vi "S8300E_reboot_UUT.vi"() -> ()   [LabVIEW 2011]
panel:
  out "Debug View":string
  out "VISA resource name out":refnum<visa-resource-name>
  out "進行狀況":string
  out "BEGIN TIME":u32
  # "2015-01-26"
  # "Error Code:MB-NG"
  # "S8300E REBOOT UUT"
  # "COM9 115200"
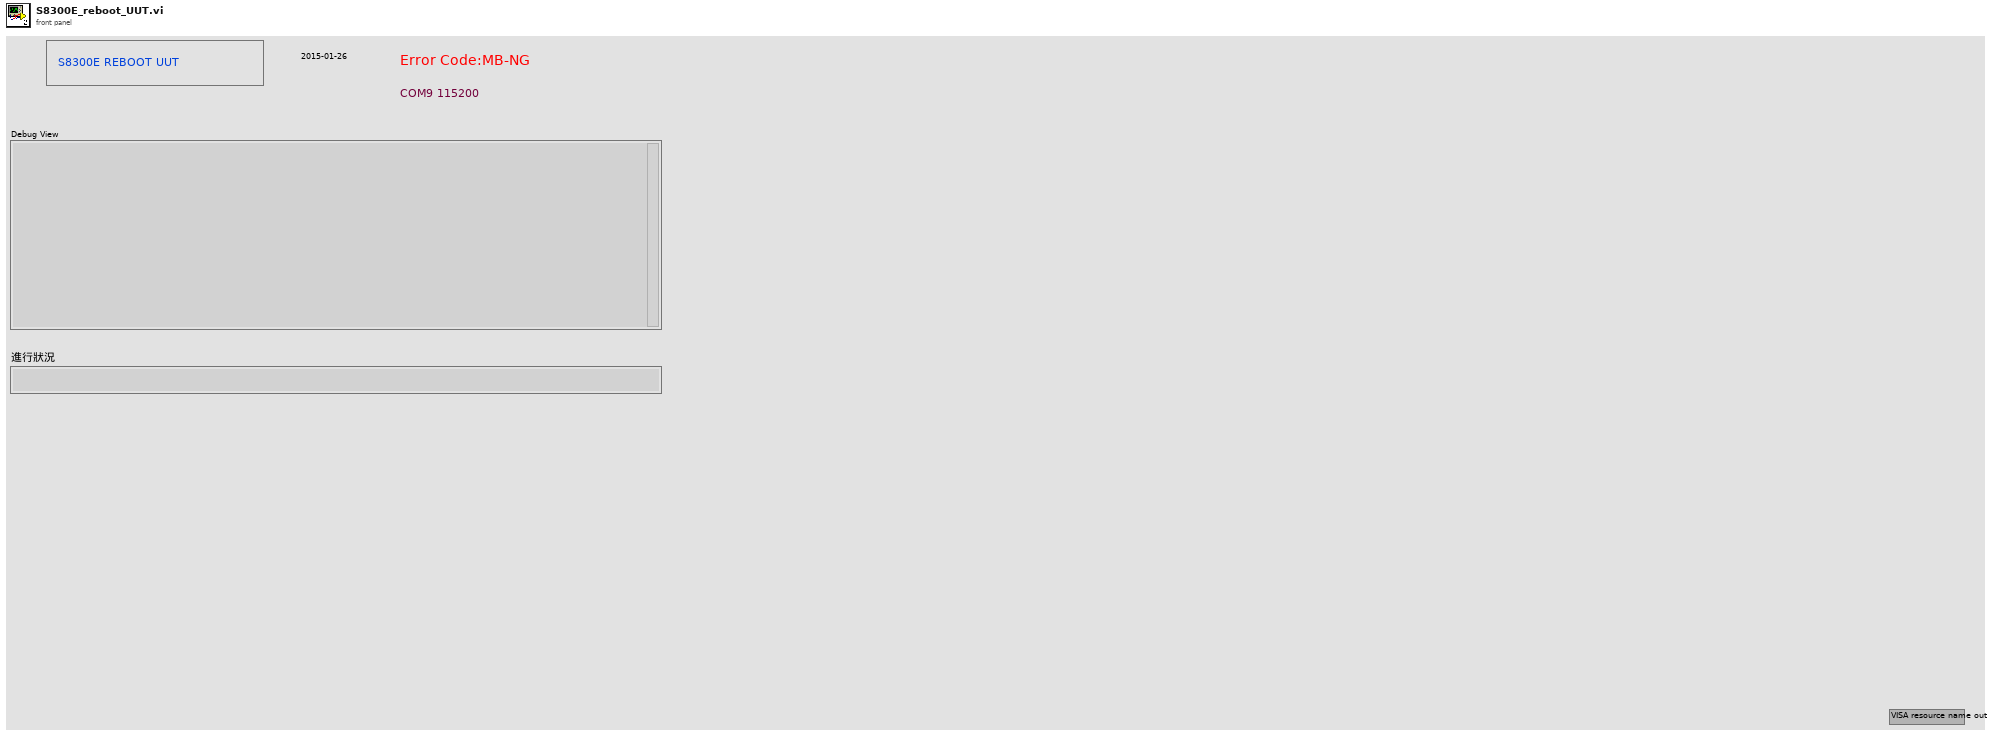
[diagram p1: front panel]
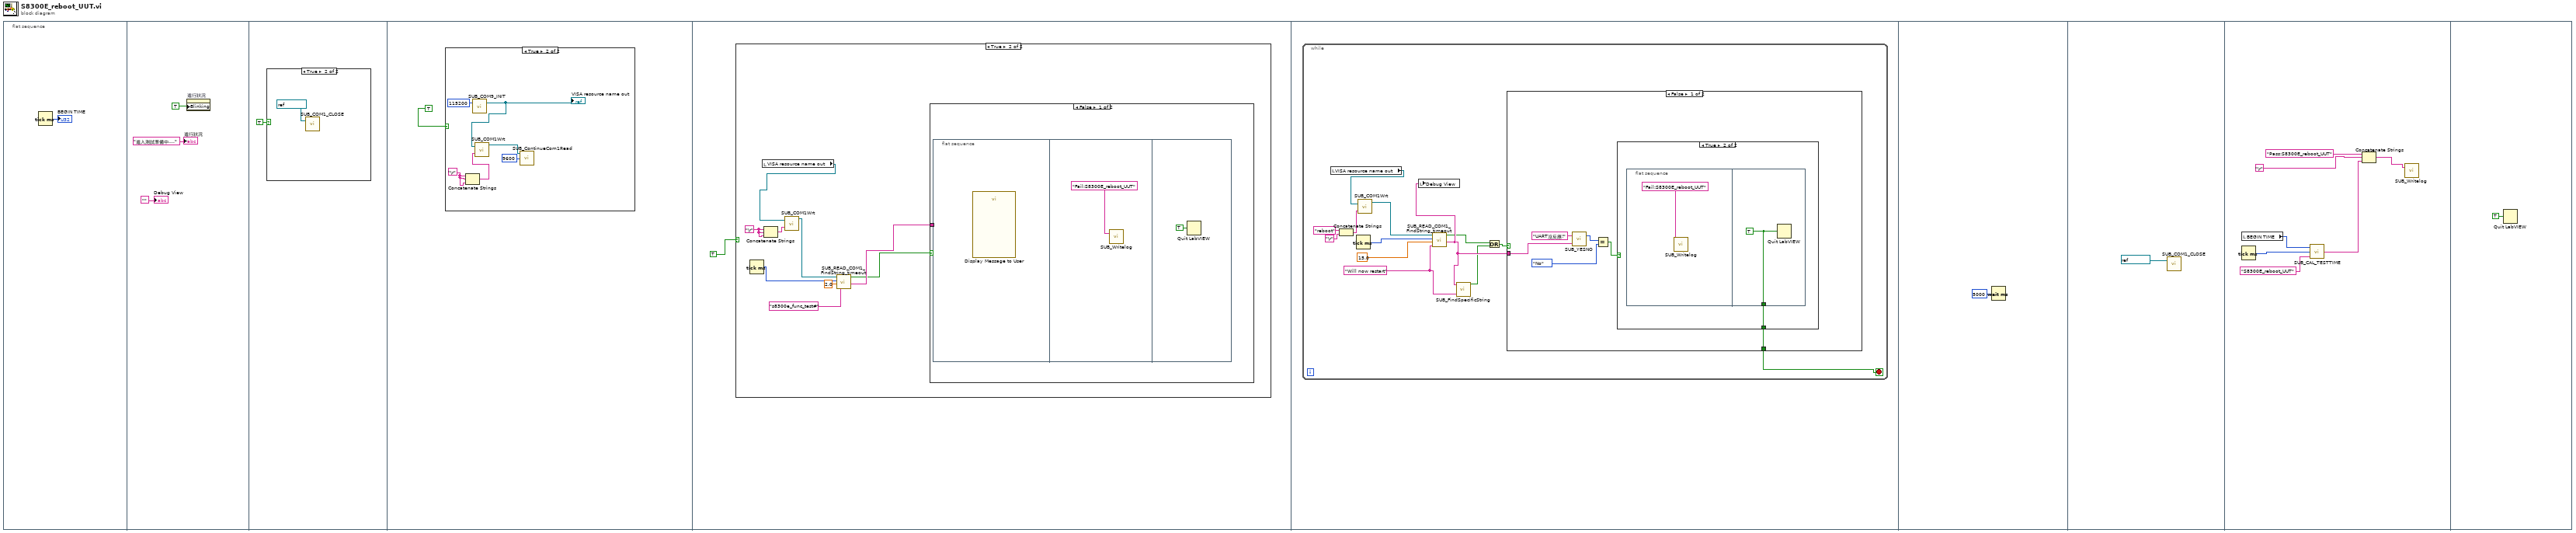
[diagram p0: block diagram]
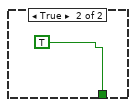
[diagram p7: hidden frame]
diagram:
  n1 = flat-sequence {
    frame #0 {
      n2 = Tick Count (ms)() -> (millisecond timer value=→"BEGIN TIME":u32)
    }
    frame #1 {
      n3 = property on="進行狀況" class="Str"("Blinking"=TRUE) -> ()  [unwired: 2 in, 2 out]
      "進行狀況" <- "進入測試準備中...." ("進行狀況")
      "Debug View" <- ""
    }
    frame #2 {
      n4 = case shown="True" TRUE {
        frame False {
        }
        frame True {
          n5 = call "SUB_COM1_CLOSE.vi"("VISA resource name"=refnum<visa-resource-name> "COM9") -> ()  [unwired: 3 in]
        }
      }
    }
    frame #3 {
      n6 = case shown="True" TRUE {
        frame False {
        }
        frame True {
          w9 = "\r"
          n7 = Concatenate Strings(w9, w9, w9) -> (w8:string)
          n8 = call "SUB_COM9_INIT.vi"("baud rate"=u32 115200) -> ("VISA resource name out"=w13:refnum<visa-resource-name>)  [unwired: 1 in, 1 out]
          "VISA resource name out" <- w13
          n9 = call "SUB_COM1Wrt.vi"("VISA resource name"=w13, "write buffer"=w8) -> ("duplicate VISA resource name"=w10:refnum<visa-resource-name>)  [unwired: 1 in, 1 out]
          n10 = call "SUB_ContinueCom1Read.vi"("Numeric"=9600, "duplicate VISA resource name 2"=w10) -> ()  [unwired: 1 in, 3 out]
        }
      }
    }
    frame #4 {
      n11 = case shown="True" TRUE {
        frame False {
        }
        frame True {
          w15 = "\r"
          n12 = Tick Count (ms)() -> (millisecond timer value=w20:u32)
          n13 = local read "VISA resource name out"() -> (w23:refnum<visa-resource-name>)
          n14 = Concatenate Strings(w15, w15, w15) -> (w16:string)
          n15 = call "SUB_COM1Wrt.vi"("VISA resource name"=w23, "write buffer"=w16) -> ("duplicate VISA resource name"=w21:refnum<visa-resource-name>)  [unwired: 1 in, 1 out]
          n16 = call "SUB_READ_COM1_FindString_timeout.vi"("Find this String"="s8300e_func_test#", "Timeout Seccond"=2.0, "Begin time"=w20, "duplicate VISA resource name 2"=w21) -> ("Output String"=w18:string, "Found String"=w17:bool)  [unwired: 1 in, 1 out]
          n17 = case shown="False" w17 {
            tunnel: w18 -> [_ _]
            frame False {
              n18 = flat-sequence {
                frame #0 {
                  n19 = call "Display Message to User"() -> ()  [unwired: 10 in, 2 out]
                }
                frame #1 {
                  n20 = call "SUB_Writelog.vi"("Pass/Fail"="Fail:S8300E_reboot_UUT") -> ()  [unwired: 2 in]
                }
                frame #2 {
                  n21 = Quit LabVIEW(quit? (T)=TRUE) -> ()
                }
              }
            }
            frame True {
            }
          }
        }
      }
    }
    frame #5 {
      n22 = while {
        stop <- w36 stop-if-true
        w29 = "Will now restart" ("Find this String")
        n23 = local read "VISA resource name out"() -> (w34:refnum<visa-resource-name>)
        n24 = Concatenate Strings("reboot" ("string"), "\r") -> (w35:string)
        n25 = Tick Count (ms)() -> (millisecond timer value=w32:u32)
        n26 = call "SUB_COM1Wrt.vi"("VISA resource name"=w34, "write buffer"=w35) -> ("duplicate VISA resource name"=w33:refnum<visa-resource-name>)  [unwired: 1 in, 1 out]
        n27 = call "SUB_READ_COM1_FindString_timeout.vi"("Find this String"=w29, "Timeout Seccond"=15.0, "Begin time"=w32, "duplicate VISA resource name 2"=w33) -> ("Output String"=w30:string, "Found String"=w27:bool)  [unwired: 1 in, 1 out]
        n28 = local write "Debug View"(w30) -> ()
        n29 = call "SUB_FindSpecificString.vi"("Find this String"=w29, "String data"=w30) -> ("Found"=w26:bool)  [unwired: 2 in, 1 out]
        n30 = Or(x=w27, y=w26) -> (x .or. y?=w28:bool)
        n31 = case shown="False" w28 {
          tunnel: [w40 TRUE] -> w36
          tunnel: w30 -> [w39 _]
          frame False {
            n32 = call "SUB_YESNO.vi"("Debug View"=w39, "Status"="UART沒反應!") -> ("yes/no"=w43:enum32{"No Selection", "Yes", "No", "None"})  [unwired: 1 in]
            n33 = Equal?(x=w43, y=enum32{"No Selection", "Yes", "No", "None"}."No") -> (x = y?=w41:bool)
            n34 = case shown="True" w41 {
              tunnel: [_ w45] -> w40
              frame False {
              }
              frame True {
                n35 = flat-sequence {
                  tunnel: [w47] -> w45
                  frame #0 {
                    n36 = call "SUB_Writelog.vi"("Pass/Fail"="Fail:S8300E_reboot_UUT") -> ()  [unwired: 2 in]
                  }
                  frame #1 {
                    w47 = TRUE ("quit? (T)")
                    n37 = Quit LabVIEW(quit? (T)=w47) -> ()
                  }
                }
              }
            }
          }
          frame True {
          }
        }
      }
    }
    frame #6 {
      n38 = Wait (ms)(milliseconds to wait=u32 5000) -> ()  [unwired: 1 out]
    }
    frame #7 {
      n39 = call "SUB_COM1_CLOSE.vi"("VISA resource name"=refnum<visa-resource-name> "COM9") -> ()  [unwired: 3 in]
    }
    frame #8 {
      n40 = Tick Count (ms)() -> (millisecond timer value=w55:u32)
      n41 = local read "BEGIN TIME"() -> (w56:u32)
      n42 = call "SUB_CAL_TESTTIME.vi"("Test Item name"="S8300E_reboot_UUT", "Stop tick time"=w55, "Start tick time"=w56) -> ("Test Time output"=w52:string)  [unwired: 2 in]
      n43 = Concatenate Strings("Pass:S8300E_reboot_UUT" ("string"), "\r", w52) -> (w51:string)
      n44 = call "SUB_Writelog.vi"("Pass/Fail"=w51) -> ()  [unwired: 2 in]
    }
    frame #9 {
      n45 = Quit LabVIEW(quit? (T)=TRUE) -> ()
    }
  }
